vi "Start Measurement.vi"(8 "error in (no error)":errorcluster, 11 "Keithley Source in":refnum<class "Keithley Source.lvclass">) -> (0 "error out":errorcluster, 3 "Keithley Source out":refnum<class "Keithley Source.lvclass">)   [LabVIEW 2015, in "Keithley Source.lvclass"]
uses:
  Keithley Source.lvclass
  Kethley Source Data.ctl
  Keithley Source.lvclass/Keithley Source.ctl
  OO Devices/Device/Read Controls Snapshot.vi
  Instrument/Read VISA Resource.vi
  Instrument/Write VISA Resource.vi
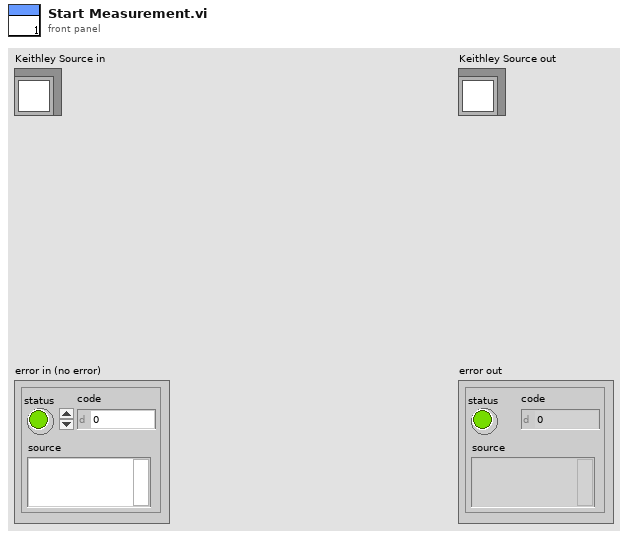
[diagram p1: front panel]
types:
  T1 = typedef "Kethley Source Data.ctl" = cluster{"Mode":enum16{"up-down sweep"}, "Start current":dbl, "End current":dbl, "Current step":dbl, "Compliance":dbl}
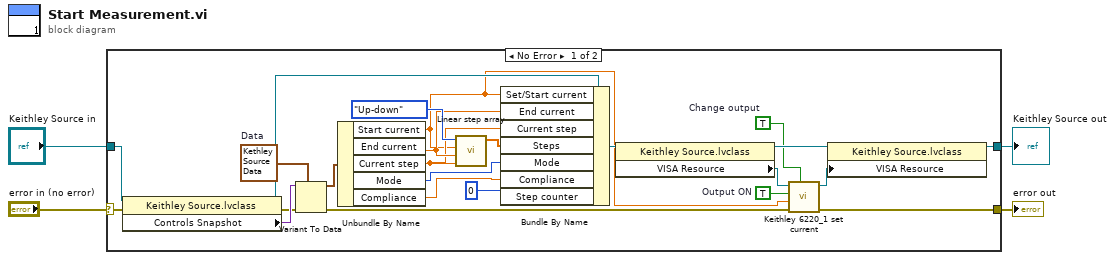
[diagram p0: block diagram]
diagram:
  n1 = case shown="No Error" "error in (no error)" {
    selector: "error in (no error)" -> [w25 w30]
    tunnel: [w10 w30] -> w3
    tunnel: [w9 w29] -> w1
    tunnel: "Keithley Source in" -> [w23 w29]
    frame No Error {
      w11 = TRUE  # Output ON
      w13 = TRUE  # Change output
      w27 = T1 {"Mode"=enum."up-down sweep", "Start current"=0.0, "End current"=0.0, "Current step"=0.0, "Compliance"=0.0}  # Data
      n2 = property class="Keithley Source.lvclass"(reference=w23, error in=w25) -> (reference out=w22:refnum<class "Keithley Source.lvclass">, error out=w26:errorcluster, "Controls Snapshot"=w28:variant)
      n3 = Variant To Data(error in=w26, type=w27, Variant=w28) -> (data=w24:T1, error out=w14:errorcluster)
      n4 = Unbundle By Name(w24) -> ("Start current"=w12:dbl, "End current"=w19:dbl, "Current step"=w18:dbl, "Mode"=w5:enum16{"up-down sweep"}, "Compliance"=w7:dbl)
      n5 = call "Linear step array.vi"("Step"=w18, "End"=w19, "Start"=w12, "Mode"=enum16{"Up", "Up-down"}."Up-down") -> ("Steps"=w17:dbl[])  [unwired: 7 in]
      n6 = Bundle By Name(cluster=w22, "Set/Start current"=w12, "End current"=w19, "Current step"=w18, "Steps"=w17, "Mode"=w5, "Compliance"=w7, "Step counter"=0) -> (w21:refnum<class "Keithley Source.lvclass">)
      n7 = property class="Keithley Source.lvclass"(reference=w21) -> (reference out=w16:refnum<class "Keithley Source.lvclass">, "VISA Resource"=w15:refnum<visa-resource-name>)  [unwired: 1 in, 1 out]
      n8 = call "Keithley 6220_1 set current.vi"("Change output"=w13, "error in (no error)"=w14, "Current (A)"=w12, "Output ON"=w11, "VISA resource name"=w15) -> ("error out"=w10:errorcluster, "VISA resource name out"=w8:refnum<visa-resource-name>)  [unwired: 5 in]
      n9 = property class="Keithley Source.lvclass"(reference=w16, "VISA Resource"=w8) -> (reference out=w9:refnum<class "Keithley Source.lvclass">)  [unwired: 1 in, 1 out]
    }
    frame Error {
    }
  }
  "error out" <- w3
  "Keithley Source out" <- w1
